vi "Reserve PWM.vi"(8 "error in (no error)":errorcluster, 9 "Purpose":string, 10 "GPIO #":T1=-1, 11 "Session in":refnum<class "Session.lvclass">) -> (0 "error out":errorcluster, 2 "PWM":refnum<class "PWM.lvclass">, 3 "Session out":refnum<class "Session.lvclass">)   [LabVIEW 2020, in "CTI.lvlib" / "Session.lvclass"]
uses:
  Session.lvclass
  GPIO Number.ctl
  PWM/PWM.lvclass
  C:/dev/cti/cti-drivers-lv-visa/CTI/Resource/Resource.lvclass
  PWM/PWM.lvclass/PWM.ctl
  GPIO/GPIO.lvclass/GPIO.ctl
  Session.lvclass/Session.ctl
  82f45d8f-1efa-45e3-b908-7d92112aac21.vi
  55ec9557-095b-406c-a094-992649bba608.vi
  82f45d8f-1efa-45e3-b908-7d92112aac21.vi/e2895f7d-be08-489f-ac40-10d6f32e0019.vi
  55ec9557-095b-406c-a094-992649bba608.vi/685f7f19-b444-4620-8f66-e6e2ddd64bb8.vi
  Generate Error.vi
  Resource/Resource.lvclass
  CTI.lvlib
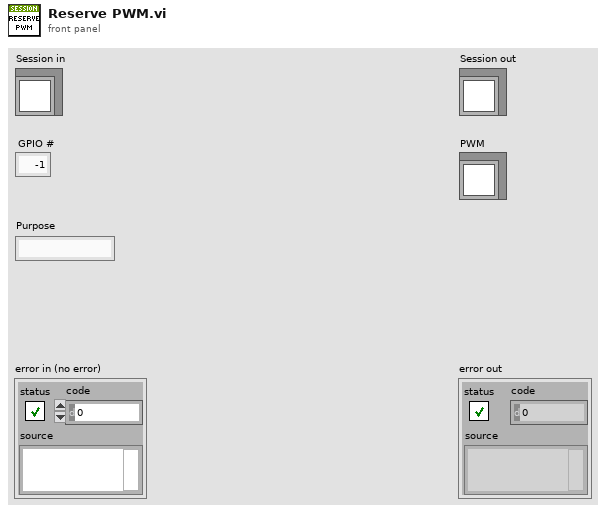
[diagram p1: front panel]
types:
  T1 = typedef "CTI.lvlib/GPIO Number.ctl" = i8
  T2 = typedef "CTI.lvlib/Session.lvclass/Resources.ctl" = cluster{"GPIO":map{T1, refnum<class "GPIO.lvclass">}, "AI":map{T3, refnum<class "AI.lvclass">}, "PWM":map{T1, refnum<class "PWM.lvclass">}, "UART":map{T4, refnum<class "UART.lvclass">}, "I2C":map{T5, refnum<class "I2C.lvclass">}, "SPI":map{T6, refnum<class "SPI.lvclass">}, "CS":map{T1, refnum<class "SPI CS.lvclass">}}
  T3 = typedef "CTI.lvlib/ADC Number.ctl" = i8
  T4 = typedef "CTI.lvlib/UART Number.ctl" = i8
  T5 = typedef "CTI.lvlib/I2C Number.ctl" = i8
  T6 = typedef "CTI.lvlib/SPI Number.ctl" = i8
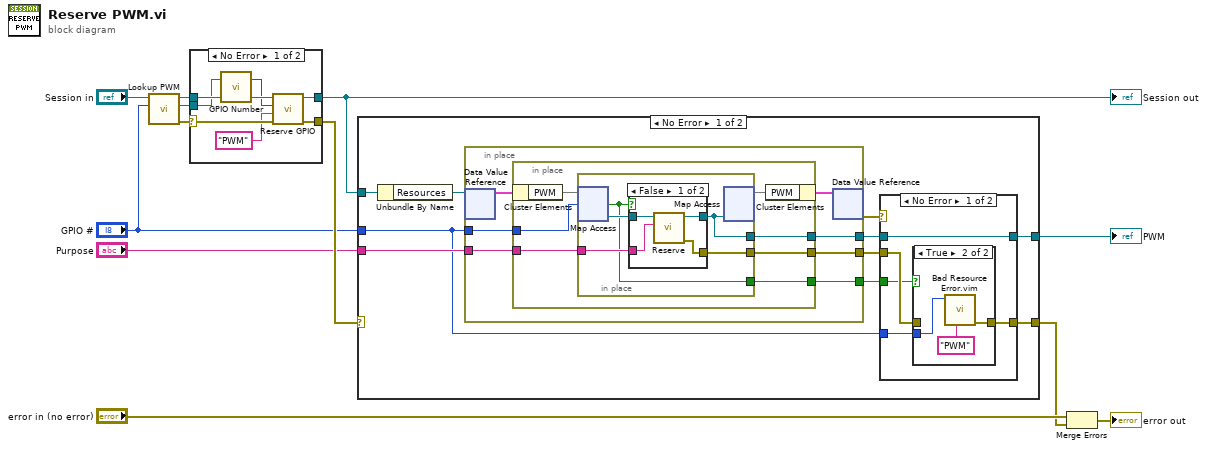
[diagram p0: block diagram]
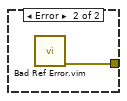
[diagram p4: hidden frame]
diagram:
  n1 = call "Lookup PWM.vi"("GPIO #"="GPIO #", "Session in"="Session in") -> ("error out"=w11:errorcluster, "PWM"=w2:refnum<class "PWM.lvclass">, "Session out"=w4:refnum<class "Session.lvclass">)  [unwired: 7 in]
  n2 = case shown="No Error" w11 {
    selector: w11 -> [w18 w20]
    tunnel: [w19 w20] -> w12
    tunnel: w4 -> [w17 w21]
    tunnel: w2 -> [w16 _]
    tunnel: [w15 w21] -> w1
    frame No Error {
      n3 = call "GPIO Number.vi"("PWM in"=w16) -> ("GPIO #"=w14:T1)  [unwired: 6 in]
      n4 = call "Reserve GPIO.vi"("error in (no error)"=w18, "Purpose"="PWM", "GPIO #"=w14, "Session in"=w17) -> ("error out"=w19:errorcluster, "Session out"=w15:refnum<class "Session.lvclass">)  [unwired: 5 in, 1 out]
    }
    frame Error {
    }
  }
  "Session out" <- w1
  n5 = case shown="No Error" w12 {
    selector: w12 -> [_ w66]
    tunnel: "Purpose" -> [w30 _]
    tunnel: [w25 _] -> w8
    tunnel: [w24 w66] -> w5
    tunnel: "GPIO #" -> [w23 _]
    tunnel: w1 -> [w22 _]
    frame No Error {
      n6 = Unbundle By Name(w22) -> ("Resources"=w31:refnum<data-value>)
      n7 = in-place {
        in-place-border: w23 -> [w48]
        in-place-border: w30 -> [w47]
        in-place-border: [w46] -> w27
        in-place-border: [w45] -> w29
        in-place-border: [w42] -> w26
        n8 = in-place-dvr #1(w31) -> (w43:T2)  [unwired: 1 out]
        n9 = in-place {
          in-place-border: w48 -> [w54]
          in-place-border: w47 -> [w53]
          in-place-border: [w52] -> w46
          in-place-border: [w51] -> w45
          in-place-border: [w49] -> w42
          n10 = in-place-cluster #2(w43) -> ("PWM"=w55:map{T1, refnum<class "PWM.lvclass">})
          n11 = in-place {
            in-place-border: w53 -> [w59]
            in-place-border: [w58] -> w51
            in-place-border: [w57] -> w52
            in-place-border: [w56] -> w49
            n12 = in-place-map #3(w55, w54) -> (w60:refnum<class "PWM.lvclass">, w57:bool)  [unwired: 1 in]
            n13 = case shown="False" w57 {
              tunnel: w60 -> [w64 w65]
              tunnel: w59 -> [w63 _]
              tunnel: [w62 w65] -> w56
              tunnel: [w61 _] -> w58
              frame False {
                n14 = call "Reserve.vi"("Purpose"=w63, "Resource in"=w64) -> ("error out"=w61:errorcluster, "Resource out"=w62:refnum<class "PWM.lvclass">)  [unwired: 8 in]
              }
              frame True {
              }
            }
            n15 = in-place-map #3(w56) -> (w50:map{T1, refnum<class "PWM.lvclass">})  [unwired: 1 in, 2 out]
          }
          n16 = in-place-cluster #2("PWM"=w50) -> (w44:T2)
        }
        n17 = in-place-dvr #1(w44) -> (w28:errorcluster)  [unwired: 1 out]
      }
      n18 = case shown="No Error" w28 {
        tunnel: w29 -> [w36 _]
        tunnel: w27 -> [w35 _]
        tunnel: [w34 w41] -> w24
        tunnel: w23 -> [w33 _]
        tunnel: w26 -> [w32 _]
        tunnel: [w32 _] -> w25
        frame No Error {
          n19 = case shown="True" w35 {
            tunnel: w36 -> [w37 _]
            tunnel: [w37 w40] -> w34
            tunnel: w33 -> [_ w39]
            frame False {
            }
            frame True {
              n20 = call "Bad Resource Error.vim"("Resource Type"="PWM", "Res #"=w39) -> ("error out"=w40:errorcluster)  [unwired: 8 in, 1 out]
            }
          }
        }
        frame Error {
          n21 = call "Bad Ref Error.vim"() -> ("error out"=w41:errorcluster)  [unwired: 10 in, 1 out]
        }
      }
    }
    frame Error {
    }
  }
  "PWM" <- w8
  n22 = Merge Errors("error in (no error)", w5) -> (→"error out":errorcluster)
